vi "Data Parser.vi"() -> ()   [LabVIEW 2018]
panel:
  out "Numeric 2":i32
  out "Numeric":i32
  in  "Input Folder":path
  in  "Output File":path
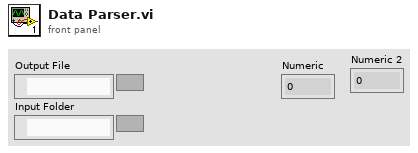
[diagram p1: front panel]
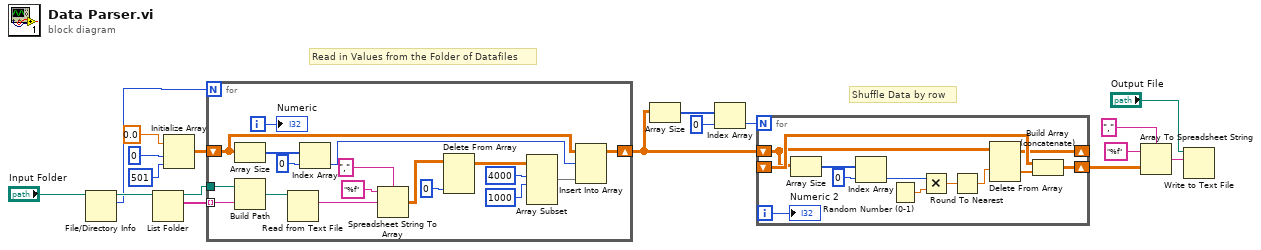
[diagram p0: block diagram]
diagram:
  # "Shuffle Data by row"
  # "Read in Values from the Folder of Datafiles"
  n1 = File/Directory Info(path="Input Folder") -> (path out=w18:path, size=w17:i64)  [unwired: 1 in, 5 out]
  n2 = List Folder(path=w18) -> (path out=w10:path, filenames=w11:string[])  [unwired: 3 in, 2 out]
  n3 = Initialize Array(0.0 ("element"), 0 ("dimension size"), 501 ("dimension size")) -> (w9:dbl[][])
  n4 = for {
    N: w17 -> [_]
    shift-right: [w20] -> w2
    shift-left: w9 -> [w24]
    tunnel: w11 -> [w27] mode=indexing
    tunnel: w10 -> [w28]
    i -> [w19]
    n5 = Array Size(array=w24) -> (size(s)=w23:i32[])
    n6 = Build Path(base path=w28, name or relative path=w27) -> (appended path=w26:path)
    n7 = Read from Text File(file (use dialog)=w26) -> (text=w36:string)  [unwired: 3 in, 3 out]
    n8 = Index Array(array=w23, index=0) -> (element=w21:i32)
    n9 = Spreadsheet String To Array(delimiter (Tab)=",", format string="%f", spreadsheet string=w36) -> (array=w33:dbl[][])  [unwired: 1 in]
    n10 = Delete From Array(array=w33, index (col)=0 ("disabled index (col)")) -> (array with subset deleted=w31:dbl[][])  [unwired: 2 in, 1 out]
    n11 = Array Subset(array=w31, index (row)=4000 ("index"), length (row)=1000 ("length")) -> (w25:dbl[][])  [unwired: 2 in]
    n12 = Insert Into Array(array=w24, index (row)=w21, new element=w25) -> (w20:dbl[][])  [unwired: 1 in]
    "Numeric" <- w19
  }
  n13 = Array Size(array=w2) -> (size(s)=w5:i32[])
  n14 = Index Array(array=w5, index=0) -> (element=w3:i32)
  n15 = for {
    N: w3 -> [_]
    shift-right: [w38] -> _
    shift-left: w2 -> [w41]
    shift-right: [w43] -> w1
    shift-left: _ -> [w42]
    i -> [w37]
    n16 = Array Size(array=w41) -> (size(s)=w48:i32[])
    n17 = Index Array(array=w48, index=0) -> (element=w45:i32)
    n18 = Random Number (0-1)() -> (number: 0 to 1=w46:dbl)
    n19 = Multiply(x=w45, y=w46) -> (x*y=w44:dbl)
    n20 = Round To Nearest(number=w44) -> (nearest integer value=w40:dbl)
    n21 = Delete From Array(array=w41, index (row)=w40) -> (deleted portion=w39:dbl[], array with subset deleted=w38:dbl[][])  [unwired: 2 in]
    n22 = Build Array (concatenate)(w42, w39) -> (w43:dbl[][])
    "Numeric 2" <- w37
  }
  n23 = Array To Spreadsheet String(delimiter (Tab)=",", array=w1, 3:"%f" ("format string")) -> (spreadsheet string=w14:string)
  n24 = Write to Text File(file (use dialog)="Output File", text=w14) -> ()  [unwired: 2 in, 3 out]
